vi "vi.ModuleExecute.vi"(0 "Module":refnum<vi>, 2 "LVCall":T1, 11 "error in":errorcluster) -> (4 "Return Data":variant, 15 "error out":errorcluster)   [LabVIEW 2014, in "GLue.lvlib" / "class.GLue.lvclass"]
uses:
  class.GLue.lvclass
  typedef.LVCallData.ctl
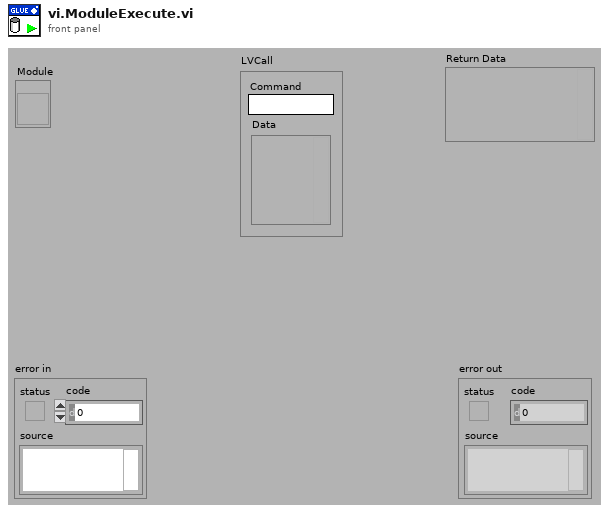
[diagram p1: front panel]
types:
  T1 = typedef "GLue.lvlib/class.GLue.lvclass/typedef.LVCallData.ctl" = cluster{"Command":string, "Data":variant}
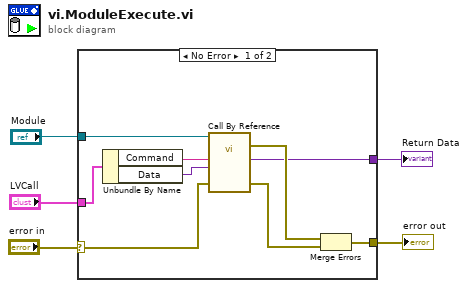
[diagram p0: block diagram]
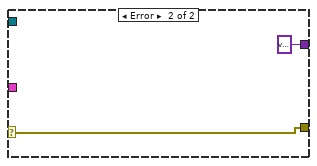
[diagram p2: hidden frame]
diagram:
  n1 = case shown="No Error" "error in" {
    selector: "error in" -> [w6 w15]
    tunnel: [w14 w15] -> w4
    tunnel: [w11 variant ("Return Data")] -> w3
    tunnel: "LVCall" -> [w9 _]
    tunnel: "Module" -> [w10 _]
    frame No Error {
      n2 = Unbundle By Name(w9) -> ("Command"=w8:string, "Data"=w7:variant)
      n3 = call-by-ref "?"(reference=w10, "error in"=w6, "Data in"=w7, "Command"=w8) -> (error out=w13:errorcluster, 0:"error out"=w12:errorcluster, "Data out"=w11:variant)  [unwired: 8 in, 1 out]
      n4 = Merge Errors(w13, w12) -> (w14:errorcluster)
    }
    frame Error {
    }
  }
  "error out" <- w4
  "Return Data" <- w3
